vi "ReadRatetest.vi"   [LabVIEW 2019]
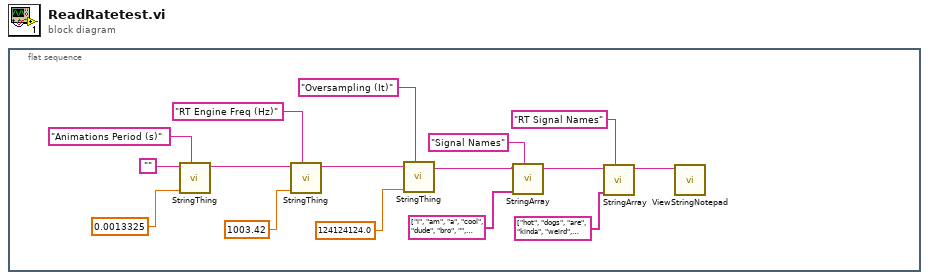
[diagram p0: block diagram]
diagram:
  n1 = flat-sequence {
    frame #0 {
      n2 = call "StringThing.vi"("Signal Name"="Animations Period (s)", "Input"=0.0013325, "Carry"="") -> ("Output"=w14:string)  [unwired: 8 in]
      n3 = call "StringThing.vi"("Signal Name"="RT Engine Freq (Hz)", "Input"=1003.42, "Carry"=w14) -> ("Output"=w12:string)  [unwired: 8 in]
      n4 = call "StringThing.vi"("Signal Name"="Oversampling (It)", "Input"=124124124.0, "Carry"=w12) -> ("Output"=w11:string)  [unwired: 8 in]
      n5 = call "StringArray.vi"("Array Name"="Signal Names", "Input"=string[] ["i", "am", "a", "cool", "dude", "bro", "", "bruh2"] ("string"), "Carry"=w11) -> ("Output"=w9:string)  [unwired: 8 in]
      n6 = call "StringArray.vi"("Array Name"="RT Signal Names", "Input"=string[] ["hot", "dogs", "are", "kinda", "weird", "yk", "", "yuh"] ("string"), "Carry"=w9) -> ("Output"=w1:string)  [unwired: 8 in]
      n7 = call "ViewStringNotepad.vi"("Input"=w1) -> ()  [unwired: 11 in]
    }
  }
